vi "highpass_image_Widefield.vi"(6 "Gauss size":i32=45, 8 "One Bulb?":bool=TRUE, 11 "Image":T1) -> (3 "high passed image":T1)   [LabVIEW 2012]
uses:
  <vilib>/vision/Image Controls.llb/IMAQ Image.ctl
  <vilib>/gmath/interp.llb/Interpolate 2D (1d xi,yi).vi
  <vilib>/vision/NI_Vision_Development_Module.lvlib
  <vilib>/gmath/NI_Gmath.lvlib
panel:
  in  "gauss21":sgl[][](array[numeric])=[[0.000334, 0.000433, 0.000547, 0.000672, 0.000803, 0.000934, 0.001056, 0.001162, 0.001245, 0.001297, 0.001315, 0.001297, 0.001245, 0.001162, 0.001056, 0.000934, 0.000803, 0.000672, 0.000547, 0.000433, 0.000334], [0.000433, 0.000562, 0.00071, 0.000872, 0.001042, 0.001211, 0.00137, 0.001508, 0.001615, 0.001682, 0.001705, 0.001682, 0.001615, 0.001508, 0.00137, 0.001211, 0.001042, 0.000872, 0.00071, 0.000562, 0.000433], [0.000547, 0.00071, 0.000896, 0.0011, 0.001315, 0.001528, 0.001729, 0.001903, 0.002038, 0.002123, 0.002152, 0.002123, 0.002038, 0.001903, 0.001729, 0.001528, 0.001315, 0.0011, 0.000896, 0.00071, 0.000547], [0.000672, 0.000872, 0.0011, 0.001351, 0.001615, 0.001877, 0.002123, 0.002337, 0.002502, 0.002607, 0.002643, 0.002607, 0.002502, 0.002337, 0.002123, 0.001877, 0.001615, 0.001351, 0.0011, 0.000872, 0.000672], [0.000803, 0.001042, 0.001315, 0.001615, 0.001929, 0.002243, 0.002537, 0.002792, 0.00299, 0.003115, 0.003158, 0.003115, 0.00299, 0.002792, 0.002537, 0.002243, 0.001929, 0.001615, 0.001315, 0.001042, 0.000803], [0.000934, 0.001211, 0.001528, 0.001877, 0.002243, 0.002607, 0.002949, 0.003246, 0.003476, 0.003621, 0.003671, 0.003621, 0.003476, 0.003246, 0.002949, 0.002607, 0.002243, 0.001877, 0.001528, 0.001211, 0.000934], [0.001056, 0.00137, 0.001729, 0.002123, 0.002537, 0.002949, 0.003336, 0.003671, 0.003931, 0.004096, 0.004153, 0.004096, 0.003931, 0.003671, 0.003336, 0.002949, 0.002537, 0.002123, 0.001729, 0.00137, 0.001056], [0.001162, 0.001508, 0.001903, 0.002337, 0.002792, 0.003246, 0.003671, 0.004041, 0.004327, 0.004508, 0.00457, 0.004508, 0.004327, 0.004041, 0.003671, 0.003246, 0.002792, 0.002337, 0.001903, 0.001508, 0.001162], [0.001245, 0.001615, 0.002038, 0.002502, 0.00299, 0.003476, 0.003931, 0.004327, 0.004633, 0.004828, 0.004894, 0.004828, 0.004633, 0.004327, 0.003931, 0.003476, 0.00299, 0.002502, 0.002038, 0.001615, 0.001245], [0.001297, 0.001682, 0.002123, 0.002607, 0.003115, 0.003621, 0.004096, 0.004508, 0.004828, 0.00503, 0.005099, 0.00503, 0.004828, 0.004508, 0.004096, 0.003621, 0.003115, 0.002607, 0.002123, 0.001682, 0.001297], [0.001315, 0.001705, 0.002152, 0.002643, 0.003158, 0.003671, 0.004153, 0.00457, 0.004894, 0.005099, 0.00517, 0.005099, 0.004894, 0.00457, 0.004153, 0.003671, 0.003158, 0.002643, 0.002152, 0.001705, 0.001315], [0.001297, 0.001682, 0.002123, 0.002607, 0.003115, 0.003621, 0.004096, 0.004508, 0.004828, 0.00503, 0.005099, 0.00503, 0.004828, 0.004508, 0.004096, 0.003621, 0.003115, 0.002607, 0.002123, 0.001682, 0.001297], [0.001245, 0.001615, 0.002038, 0.002502, 0.00299, 0.003476, 0.003931, 0.004327, 0.004633, 0.004828, 0.004894, 0.004828, 0.004633, 0.004327, 0.003931, 0.003476, 0.00299, 0.002502, 0.002038, 0.001615, 0.001245], [0.001162, 0.001508, 0.001903, 0.002337, 0.002792, 0.003246, 0.003671, 0.004041, 0.004327, 0.004508, 0.00457, 0.004508, 0.004327, 0.004041, 0.003671, 0.003246, 0.002792, 0.002337, 0.001903, 0.001508, 0.001162], [0.001056, 0.00137, 0.001729, 0.002123, 0.002537, 0.002949, 0.003336, 0.003671, 0.003931, 0.004096, 0.004153, 0.004096, 0.003931, 0.003671, 0.003336, 0.002949, 0.002537, 0.002123, 0.001729, 0.00137, 0.001056], [0.000934, 0.001211, 0.001528, 0.001877, 0.002243, 0.002607, 0.002949, 0.003246, 0.003476, 0.003621, 0.003671, 0.003621, 0.003476, 0.003246, 0.002949, 0.002607, 0.002243, 0.001877, 0.001528, 0.001211, 0.000934], [0.000803, 0.001042, 0.001315, 0.001615, 0.001929, 0.002243, 0.002537, 0.002792, 0.00299, 0.003115, 0.003158, 0.003115, 0.00299, 0.002792, 0.002537, 0.002243, 0.001929, 0.001615, 0.001315, 0.001042, 0.000803], [0.000672, 0.000872, 0.0011, 0.001351, 0.001615, 0.001877, 0.002123, 0.002337, 0.002502, 0.002607, 0.002643, 0.002607, 0.002502, 0.002337, 0.002123, 0.001877, 0.001615, 0.001351, 0.0011, 0.000872, 0.000672], [0.000547, 0.00071, 0.000896, 0.0011, 0.001315, 0.001528, 0.001729, 0.001903, 0.002038, 0.002123, 0.002152, 0.002123, 0.002038, 0.001903, 0.001729, 0.001528, 0.001315, 0.0011, 0.000896, 0.00071, 0.000547], [0.000433, 0.000562, 0.00071, 0.000872, 0.001042, 0.001211, 0.00137, 0.001508, 0.001615, 0.001682, 0.001705, 0.001682, 0.001615, 0.001508, 0.00137, 0.001211, 0.001042, 0.000872, 0.00071, 0.000562, 0.000433], [0.000334, 0.000433, 0.000547, 0.000672, 0.000803, 0.000934, 0.001056, 0.001162, 0.001245, 0.001297, 0.001315, 0.001297, 0.001245, 0.001162, 0.001056, 0.000934, 0.000803, 0.000672, 0.000547, 0.000433, 0.000334]] format="%0.3f"
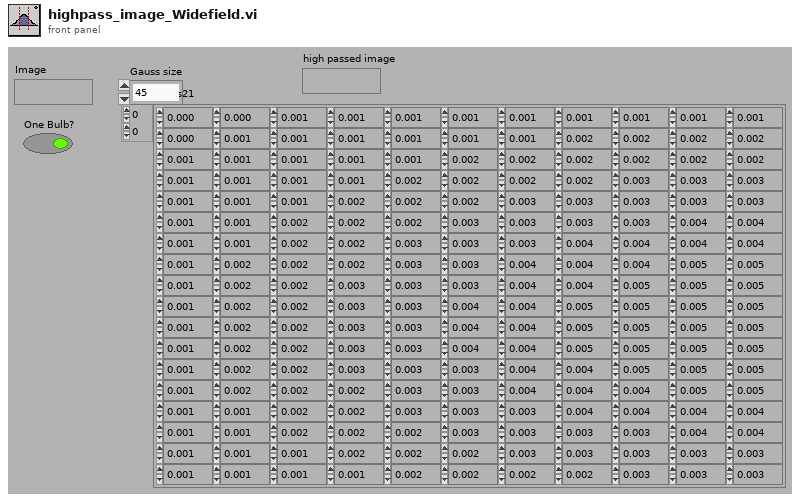
[diagram p1: front panel]
types:
  T1 = typedef "IMAQ Image.ctl" = refnum<image>
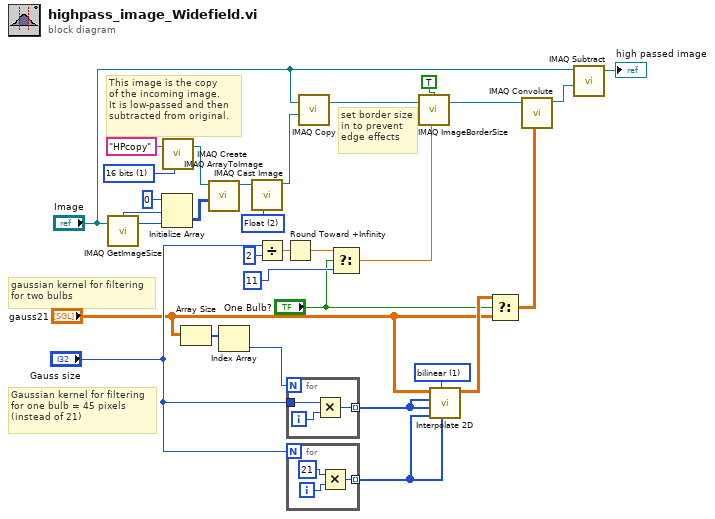
[diagram p0: block diagram]
diagram:
  w15 = 1 items=["nearest", "bilinear", "bicubic", "bicubic spline"] ("method")
  w9 = u32 2 items=["8 bits", "16 bits", "Float", "Complex", "RGB", "HSL"] ("Image Type")
  w29 = u32 1 items=["8 bits", "16 bits", "Float", "Complex", "RGB", "HSL"] ("Image Type")
  # "gaussian kernel for filtering\nfor two bulbs"
  # "Gaussian kernel for filtering\nfor one bulb = 45 pixels\n(instead of 21)"
  # "set border size\nin to prevent\nedge effects"
  # "This image is the copy \nof the incoming image. \nIt is low-passed and then\nsubtracted from original."
  n1 = call "IMAQ GetImageSize"("Image"="Image") -> ("Y Resolution"=w26:i32, "X Resolution"=w25:i32)  [unwired: 1 in, 3 out]
  n2 = Initialize Array(0, w25, w26) -> (w28:i32[][])
  n3 = call "IMAQ Create"("Image Name"="HPcopy", "Image Type"=w29) -> ("New Image"=w30:T1)  [unwired: 2 in, 2 out]
  n4 = Array Size(array="gauss21") -> (size(s)=w2:i32[])
  n5 = call "IMAQ ArrayToImage"("Image Pixels (I16)"=w28, "Image"=w30) -> ("Image Out"=w27:T1)  [unwired: 4 in, 5 out]
  n6 = Index Array(array=w2) -> (element=w1:i32)  [unwired: 1 in]
  n7 = call "IMAQ Cast Image"("Image Type"=w9, "Image Src"=w27) -> ("Image Dst Out"=w23:T1)  [unwired: 4 in, 5 out]
  n8 = Divide(x="Gauss size", y=2) -> (x/y=w7:dbl)
  n9 = Round Toward +Infinity(x=w7) -> (ceil(x): smallest int >= x=w5:dbl)
  n10 = for {
    N: w1 -> [_]
    tunnel: [w33] -> w14 mode=indexing
    tunnel: "Gauss size" -> [w32]
    i -> [w34]
    n11 = Multiply(x=w32, y=w34) -> (x*y=w33:i32)
  }
  n12 = for {
    N: "Gauss size" -> [_]
    tunnel: [w35] -> w13 mode=indexing
    i -> [w37]
    n13 = Multiply(x=21, y=w37) -> (x*y=w35:i32)
  }
  n14 = call "IMAQ Copy"("Image Dst"=w23, "Image Src"="Image") -> ("Image Dst Out"=w19:T1)  [unwired: 1 in, 4 out]
  n15 = Select(t=w5, s="One Bulb?", f=11 ("Image border size in")) -> (s? t:f=w11:dbl)
  n16 = call "IMAQ ImageBorderSize"("Get/Set Status? (Set)"=TRUE, "Image"=w19, "Image border size in"=w11) -> ("Image Out"=w18:T1)  [unwired: 1 in, 2 out]
  n17 = call-poly <vilib>:"Interpolate 2D.vi"("yi"=w13, "method"=w15, "xi"=w13, "Y"=w14, "X"=w14, "Z"="gauss21") -> ("zi"=w12:dbl[][])  [unwired: 1 in, 4 out]
  n18 = Select(t=w12, s="One Bulb?", f="gauss21") -> (s? t:f=w16:dbl[][])
  n19 = call "IMAQ Convolute"("Kernel"=w16, "Image Src"=w18) -> ("Image Dst Out"=w21:T1)  [unwired: 5 in, 4 out]
  n20 = call "IMAQ Subtract"("Image Src A"="Image", "Image Src B"=w21) -> ("Image Dst Out"=→"high passed image":T1)  [unwired: 3 in, 3 out]
